vi "Host.vi"() -> ()   [LabVIEW 2025]
uses:
  <vilib>/FPGAPlugInAG/cRIO-9035/niLvFpga_Open_cRIO-9035.vi
  <vilib>/rvi/interface/common/dynamic/niFpgaDynamicAddResources.vi
  <vilib>/FPGAPlugInAG/Dynamic/niLvFpga_Reset_Dynamic.vi
  <vilib>/Utility/error.llb/Error Cluster From Error Code.vi
  <vilib>/rvi/errors/niLvFpgaAdjustHostInterfaceError.vi
  <vilib>/FPGAPlugInAG/Dynamic/niLvFpga_Run_Dynamic.vi
  <vilib>/FPGAPlugInAG/Dynamic/niLvFpga_Close_Dynamic.vi
  <vilib>/rvi/interface/nirviOpenFPGA/nirviOpenFPGA.xnode
  FPGA Bitfiles/kintex7timing_FPGATarget_Target_3m86y6BdVqo.lvbitx
  <vilib>/rvi/interface/nirviMethod/nirviMethod.xnode
  <vilib>/rvi/interface/nirviCloseFPGA/nirviCloseFPGA.xnode
  <vilib>/rvi/errors/niLvFpgaMergeErrorWithErrorCode.vi
  <vilib>/FPGAPlugInAG/Dynamic/niLvFpga_WriteFifo_Dynamic.vi
  <vilib>/FPGAPlugInAG/Dynamic/niLvFpga_ReadFifo_Dynamic.vi
panel:
  out "x-y":dbl
  out "Data":u32[](array[numeric])
  out "Numeric":i32
  out "Controlled Force":sgl[](graph)
  out "Uncontrolled Displacement":dynamicdata(graph)
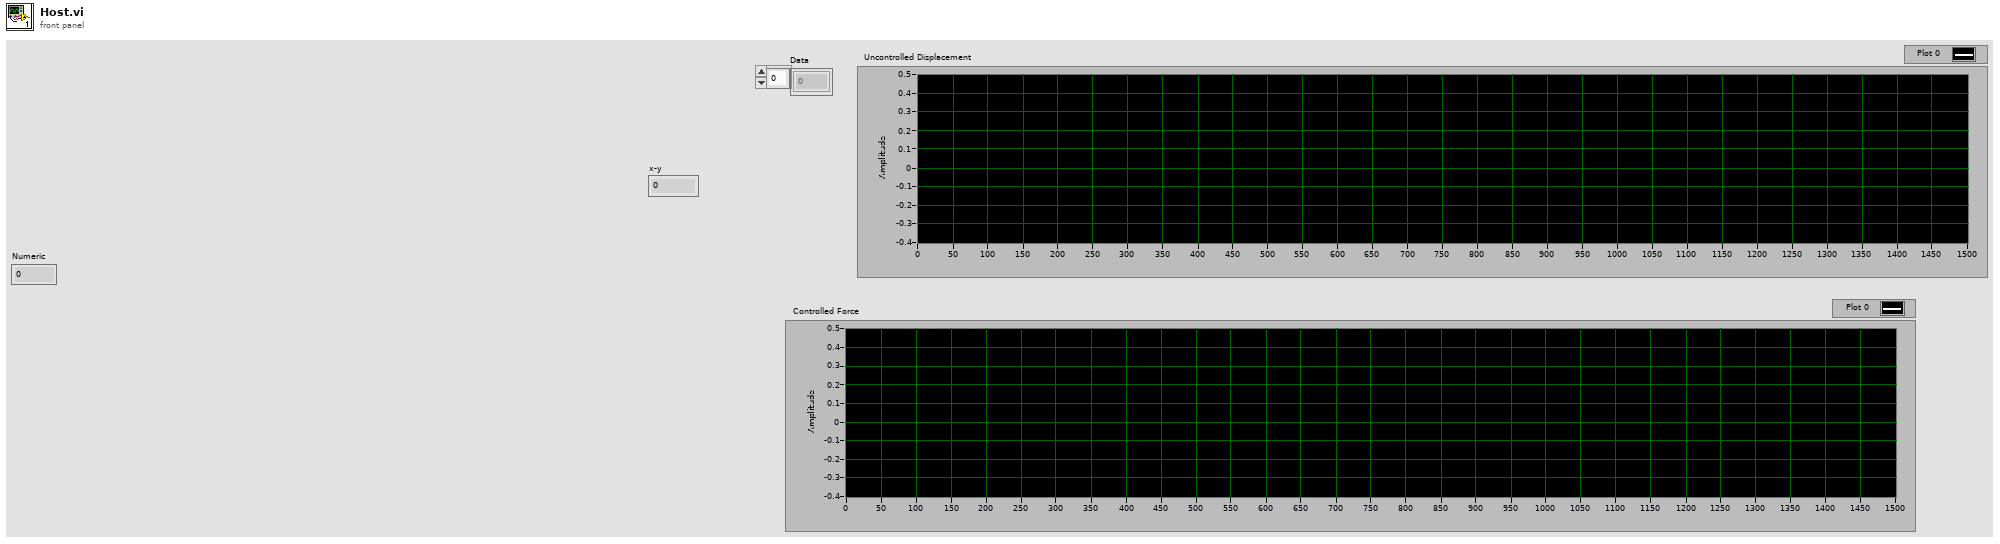
[diagram p1: front panel]
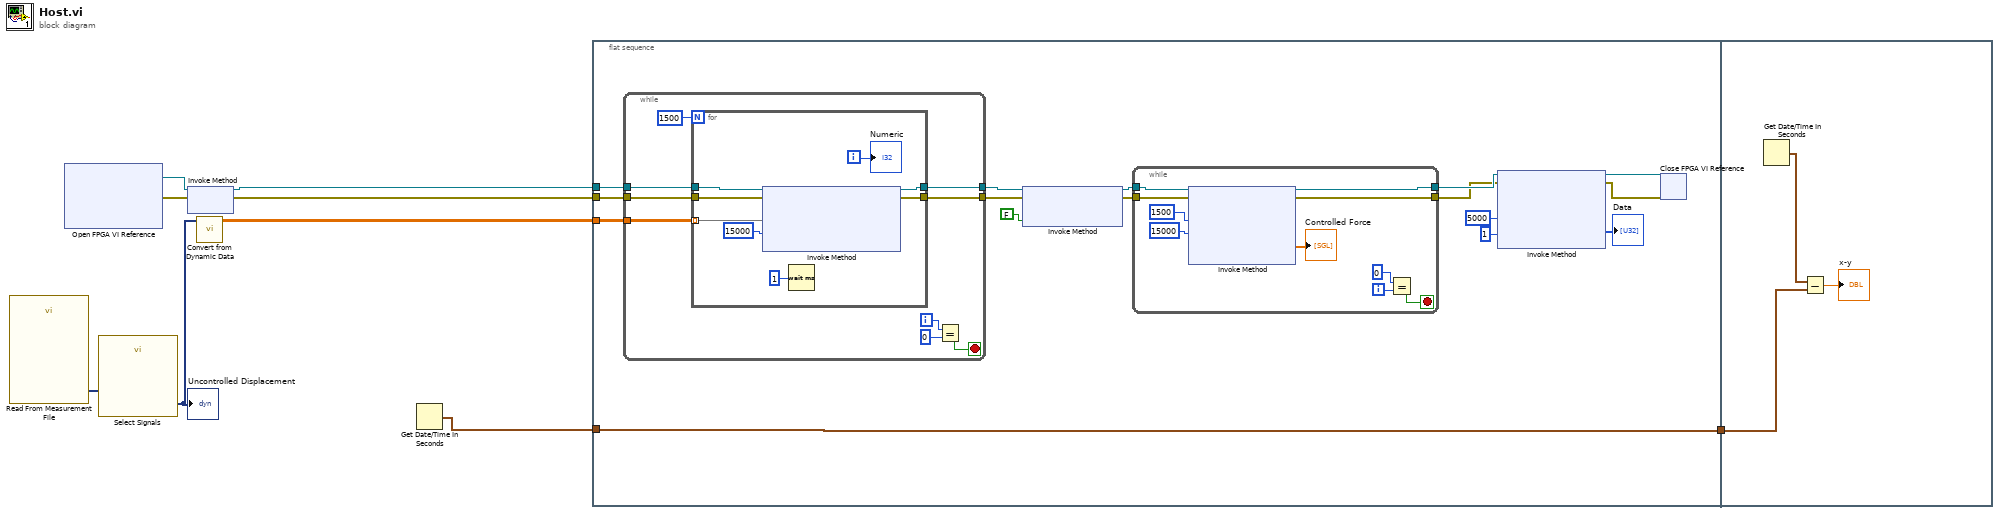
[diagram p0: block diagram]
diagram:
  n1 = call "Read From Measurement File"() -> ("Signals"=w9:dynamicdata)  [unwired: 6 in, 5 out]
  n2 = xnode "Open FPGA VI Reference"() -> ("FPGA VI Reference Out"=w6:refnum<k20>, "error out"=w4:errorcluster)  [unwired: 2 in]
  n3 = call "Select Signals"("Signals"=w9) -> ("Signal Out"=w8:dynamicdata)  [unwired: 9 in, 1 out]
  "Uncontrolled Displacement" <- w8
  n4 = xnode "Invoke Method"("FPGA VI Reference In"=w6, "error in"=w4) -> ("FPGA VI Reference Out"=w5:refnum<k20>, "error out"=w3:errorcluster)
  n5 = call "Convert from Dynamic Data"("Dynamic Data Type"=w8) -> ("Array"=w7:dbl[][])  [unwired: 3 in]
  n6 = Get Date/Time In Seconds() -> (seconds since 1Jan1904=w1:timestamp)
  n7 = flat-sequence {
    tunnel: w7 -> [w25]
    tunnel: w5 -> [w24]
    tunnel: w3 -> [w20]
    tunnel: [w10] -> w2
    tunnel: w1 -> [w10]
    tunnel: w2 -> [w54]
    frame #0 {
      n8 = while {
        tunnel: w25 -> [w33]
        tunnel: w24 -> [w32]
        tunnel: [w30] -> w23
        tunnel: w20 -> [w27]
        tunnel: [w26] -> w19
        i -> [w28]
        stop <- w31 stop-if-true
        n9 = for {
          N: 1500 -> [_]
          tunnel: w33 -> [w39] mode=indexing
          tunnel: w32 -> [w40]
          tunnel: [w38] -> w30
          tunnel: w27 -> [w36]
          tunnel: [w35] -> w26
          i -> [w37]
          n10 = xnode "Invoke Method"("FPGA VI Reference In"=w40, "error in"=w36, "Data"=w39, "Timeout (ms)"=15000) -> ("FPGA VI Reference Out"=w38:refnum<k20>, "error out"=w35:errorcluster)  [unwired: 1 out]
          n11 = Wait (ms)(milliseconds to wait=u32 1) -> ()  [unwired: 1 out]
          "Numeric" <- w37
        }
        n12 = Equal?(x=w28, y=u32 0) -> (x = y?=w31:bool)
      }
      n13 = xnode "Invoke Method"("FPGA VI Reference In"=w23, "error in"=w19, "Wait Until Done (F)"=FALSE) -> ("FPGA VI Reference Out"=w22:refnum<k20>, "error out"=w18:errorcluster)
      n14 = while {
        tunnel: [w51] -> w14
        tunnel: w22 -> [w49]
        tunnel: w18 -> [w44]
        tunnel: [w43] -> w13
        i -> [w48]
        stop <- w46 stop-if-true
        n15 = xnode "Invoke Method"("FPGA VI Reference In"=w49, "error in"=w44, "Number of Elements"=u32 1500, "Timeout (ms)"=15000) -> ("FPGA VI Reference Out"=w51:refnum<k20>, "error out"=w43:errorcluster, "Data"=→"Controlled Force":sgl[])  [unwired: 1 out]
        n16 = Equal?(x=0, y=w48) -> (x = y?=w46:bool)
      }
      n17 = xnode "Invoke Method"("FPGA VI Reference In"=w14, "error in"=w13, "Number of Elements"=u32 1, "Timeout (ms)"=5000) -> ("FPGA VI Reference Out"=w12:refnum<k20>, "error out"=w11:errorcluster, "Data"=→"Data":u32[])  [unwired: 1 out]
      n18 = xnode "Close FPGA VI Reference"("FPGA VI Reference In"=w12, "error in"=w11) -> ()  [unwired: 1 out]
    }
    frame #1 {
      n19 = Get Date/Time In Seconds() -> (seconds since 1Jan1904=w55:timestamp)
      n20 = Subtract(x=w55, y=w54) -> (x-y=→"x-y":dbl)
    }
  }
